vi "Function.vi"(8 "error in (no error)":errorcluster, 9 "Numeric B":csg, 10 "Numeric A":csg, 11 "Two Terminal in":refnum<class "Less_CPLX_SGL.lvclass">) -> (0 "error out":errorcluster, 2 "Result":bool, 3 "Two Terminal out":refnum<class "Less_CPLX_SGL.lvclass">)   [LabVIEW 2021, in "Less_CPLX_SGL.lvclass"]
uses:
  Less_CPLX_SGL.lvclass
  Less_CPLX_SGL.lvclass/Less_CPLX_SGL.ctl
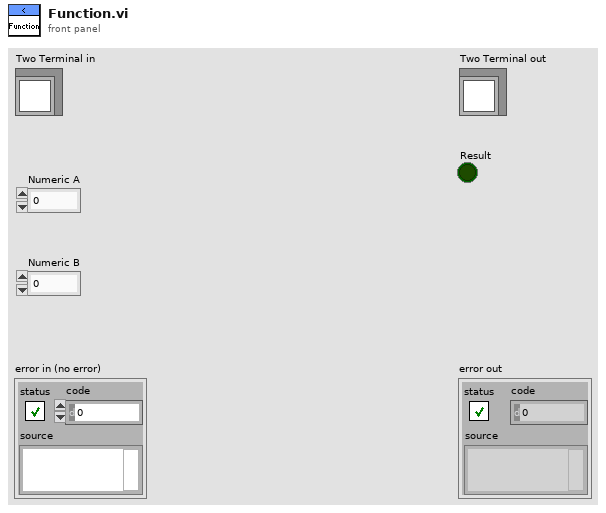
[diagram p1: front panel]
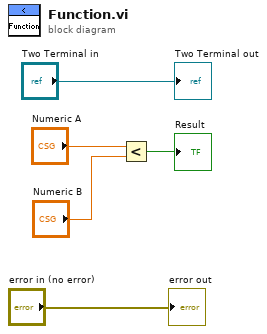
[diagram p0: block diagram]
diagram:
  n1 = Less?(x="Numeric A", y="Numeric B") -> (x < y?=→"Result":bool)
  "error out" <- "error in (no error)"
  "Two Terminal out" <- "Two Terminal in"
